vi "DSF.Engine.Memory.Cache.Get Transfers Groups.vi"(11 "Cache in":refnum<class "DSF.Engine.Memory.Cache.lvclass">) -> (2 "Transfers Groups":refnum<class "DSF.Engine.Transfer Group.lvclass">[](array[class]), 3 "Cache out":refnum<class "DSF.Engine.Memory.Cache.lvclass">)   [LabVIEW 2017, in "Data Sharing Framework Engine.lvlib" / "DSF.Engine.Memory.Cache.lvclass"]
uses:
  DSF.Engine.Memory.Cache.lvclass
  Transfer/DSF.Engine.Transfer Group.lvclass
  DSF.Engine.Memory.Cache.lvclass/DSF.Engine.Memory.Cache.ctl
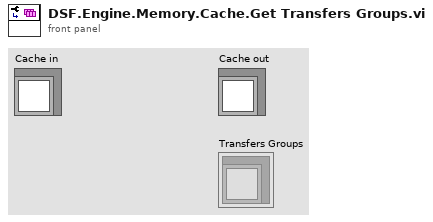
[diagram p1: front panel]
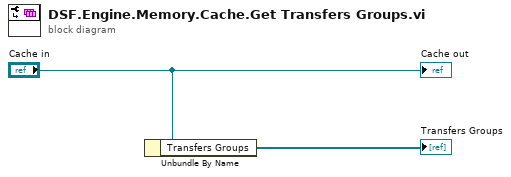
[diagram p0: block diagram]
diagram:
  n1 = Unbundle By Name("Cache in") -> ("Transfers Groups"=→"Transfers Groups":refnum<class "DSF.Engine.Transfer Group.lvclass">[])
  "Cache out" <- "Cache in"
